vi "discrete_control_memory.vi"() -> ()   [LabVIEW 2019]
panel:
  out "integral_error":dbl
  out "w_d[k]":dbl
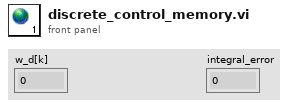
[diagram p1: front panel]
diagram:
